vi "ep_Linear Interpolate.vi"(8 "y2":dbl format="%.2f", 9 "y1":dbl format="%.2f", 10 "x2":dbl format="%.2f", 11 "x1":dbl format="%.2f") -> (3 "y":dbl format="%.6f")   [LabVIEW 2011, in "NI_EP_Power Quality.lvlib"]
uses:
  <vilib>/addons/Electrical Power/PQ/NI_EP_Power Quality.lvlib
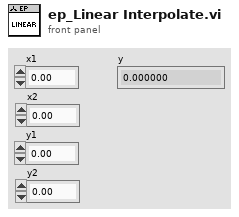
[diagram p1: front panel]
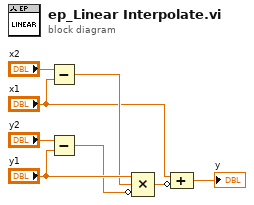
[diagram p0: block diagram]
diagram:
  n1 = Subtract(x="x2", y="x1") -> (x-y=w5:dbl)
  n2 = Subtract(x="y2", y="y1") -> (x-y=w4:dbl)
  n3 = Compound Arithmetic op=MULTIPLY("y1", w5, invert w4) -> (w3:dbl)
  n4 = Compound Arithmetic op=ADD("x1", invert w3) -> (→"y":dbl)
